vi "AES-Single-Round-Top.vi"(9 "state (_c) U64":u64[](array[numeric]) format="%.0x", 11 "key (_a)":u64[](array[numeric]) format="%.0x") -> (1 "state out (c) U64":u64[](array[numeric]) format="%.0x")   [LabVIEW 2017]
uses:
  AES-xtime.vi
panel:
  out "ADD_KEY":u8[](array[numeric]) format="%.0x"
  out "MIX_COLUMNS":u8[](array[numeric]) format="%.0x"
  out "SHIFT_ROWS":u8[](array[numeric]) format="%.0x"
  out "SUB_BYTES":u8[](array[numeric]) format="%.0x"
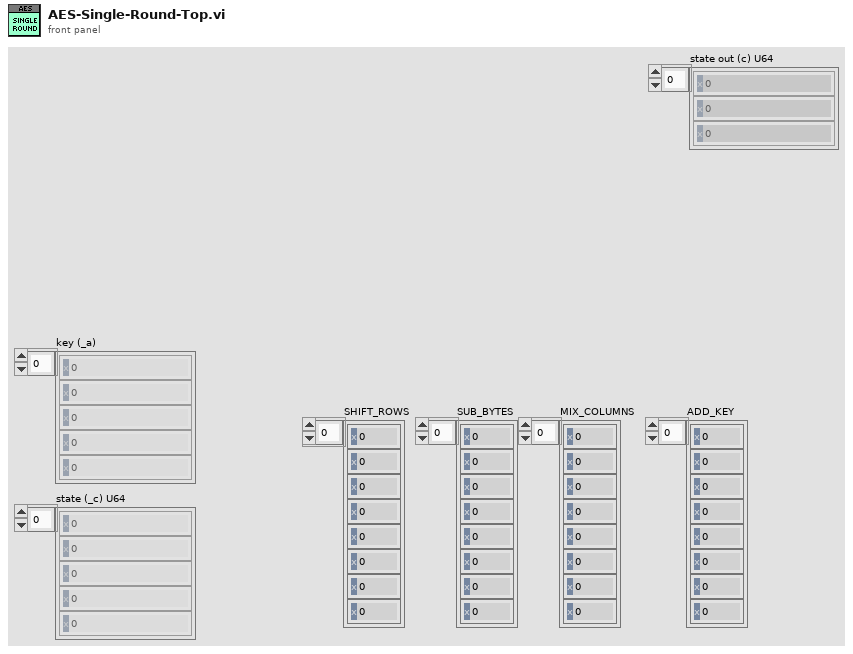
[diagram p1: front panel]
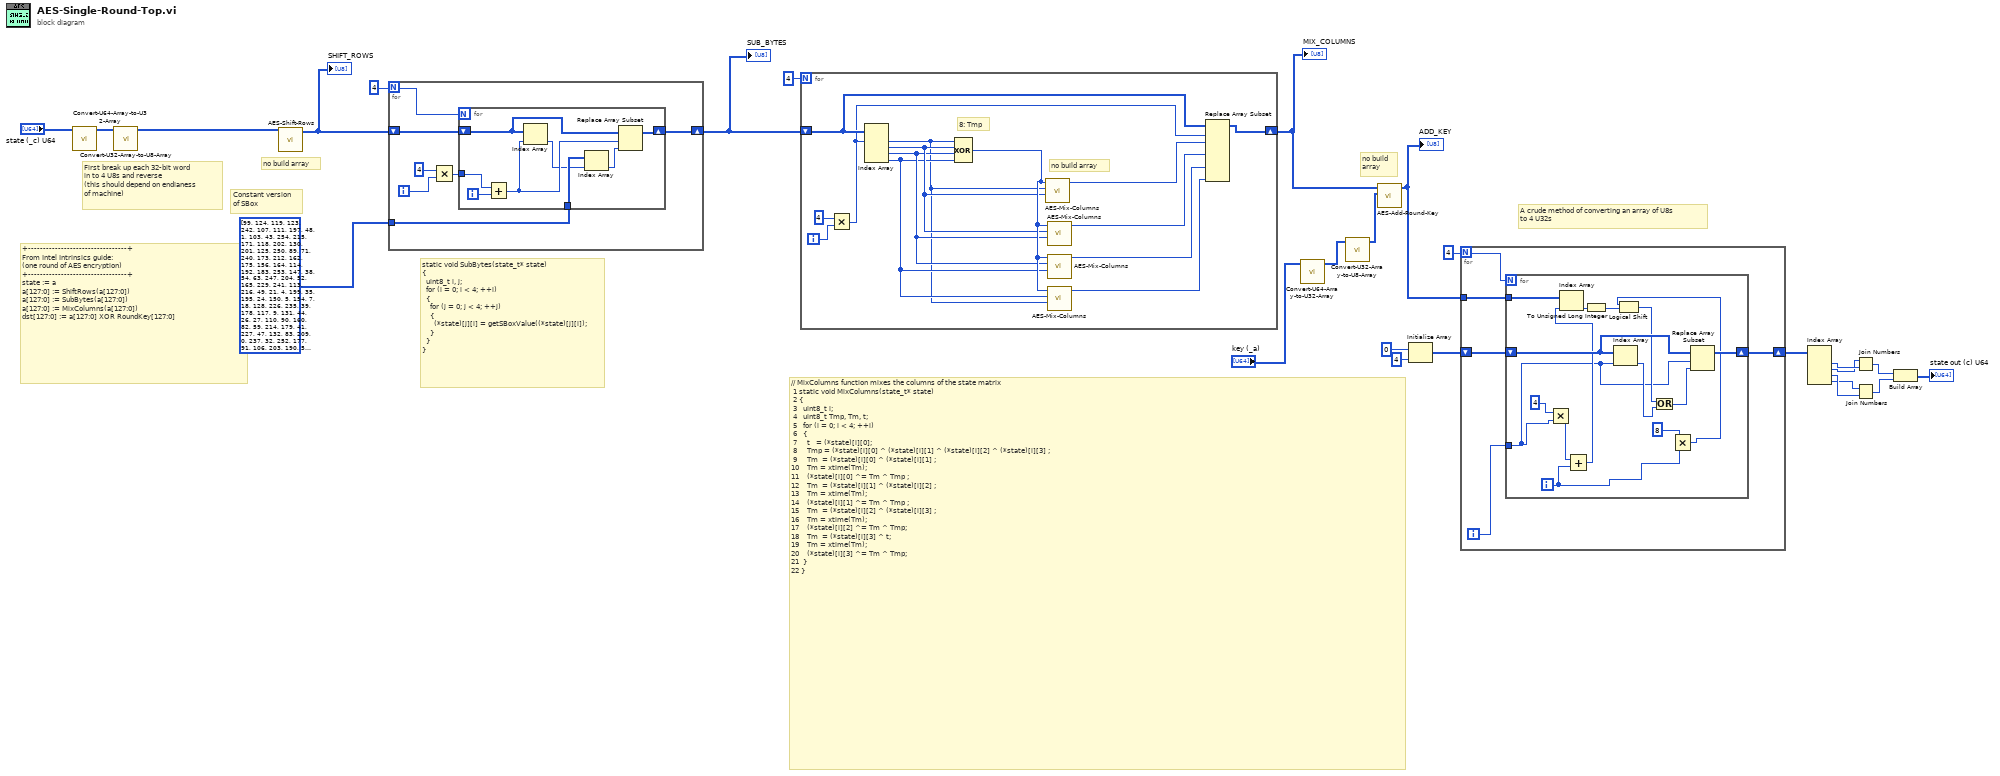
[diagram p0: block diagram]
diagram:
  # "A crude method of converting an array of U8s\nto 4 U32s"
  # "no build\narray"
  # "no build array"
  # "Constant version\nof SBox"
  # "// MixColumns function mixes the columns of the state matrix\n 1 static void MixColumns(state_t* state)\n 2 {\n 3   uint8_t i;\n 4   uint8_t Tmp, Tm, t;\n 5   for (i = 0; i < 4; ++i)\n 6   {  \n 7     t   = (*state)[i][0]; \n 8     Tmp = (*state)[i][0] ^ (*state)[i][1] ^ (*state)[i][2] ^ (*state)[i][3] ;\n 9     Tm  = (*state)[i][0] ^ (*state)[i][1] ;\n10    Tm = xtime(Tm);  \n11    (*state)[i][0] ^= Tm ^ Tmp ;\n12    Tm  = (*state)[i][1] ^ (*state)[i][2] ; \n13    Tm = xtime(Tm);  \n14    (*state)[i][1] ^= Tm ^ Tmp ;\n15    Tm  = (*state)[i][2] ^ (*state)[i][3] ;\n16    Tm = xtime(Tm);\n17    (*state)[i][2] ^= Tm ^ Tmp;\n18    Tm  = (*state)[i][3] ^ t;\n19    Tm = xtime(Tm);\n20    (*state)[i][3] ^= Tm ^ Tmp;\n21  }\n22 }"
  # "static void SubBytes(state_t* state)\n{\n  uint8_t i, j;\n  for (i = 0; i < 4; ++i)\n  {\n    for (j = 0; j < 4; ++j)\n    {\n      (*state)[j][i] = getSBoxValue((*state)[j][i]);\n    }\n  }\n}"
  # "First break up each 32-bit word\nin to 4 U8s and reverse\n(this should depend on endianess\nof machine)"
  # "+---------------------------------+\nFrom Intel Intrinsics guide:\n(one round of AES encryption)\n+---------------------------------+\nstate := a\na[127:0] := ShiftRows(a[127:0])\na[127:0] := SubBytes(a[127:0])\na[127:0] := MixColumns(a[127:0])\ndst[127:0] := a[127:0] XOR RoundKey[127:0]"
  n1 = call "Convert-U64-Array-to-U32-Array.vi"("2 x U64"="state (_c) U64") -> ("4 x U32"=w9:u32[])  [unwired: 10 in]
  n2 = call "Convert-U32-Array-to-U8-Array.vi"("state"=w9) -> ("Array"=w25:u8[])  [unwired: 10 in]
  n3 = call "AES-Shift-Rows.vi"("Data In"=w25) -> ("Data Out"=w23:u8[])  [unwired: 10 in]
  "SHIFT_ROWS" <- w23
  n4 = for {
    N: 4 -> [w32]
    shift-right: [w29] -> w21
    shift-left: w23 -> [w31]
    tunnel: u8[] [99, 124, 119, 123, 242, 107, 111, 197, 48, 1, 103, 43, 254, 215, 171, 118, 202, 130, 201, 125, 250, 89, 71, 240, 173, 212, 162, 175, 156, 164, 114, 192, 183, 253, 147, 38, 54, 63, 247, 204, 52, 165, 229, 241, 113, 216, 49, 21, 4, 199, 35, 195, 24, 150, 5, 154, 7, 18, 128, 226, 235, 39, 178, 117, 9, 131, 44, 26, 27, 110, 90, 160, 82, 59, 214, 179, 41, 227, 47, 132, 83, 209, 0, 237, 32, 252, 177, 91, 106, 203, 190, 57, 74, 76, 88, 207, 208, 239, 170, 251, 67, 77, 51, 133, 69, 249, 2, 127, 80, 60, 159, 168, 81, 163, 64, 143, 146, 157, 56, 245, 188, 182, 218, 33, 16, 255, 243, 210, 205, 12, 19, 236, 95, 151, 68, 23, 196, 167, 126, 61, 100, 93, 25, 115, 96, 129, 79, 220, 34, 42, 144, 136, 70, 238, 184, 20, 222, 94, 11, 219, 224, 50, 58, 10, 73, 6, 36, 92, 194, 211, 172, 98, 145, 149, 228, 121, 231, 200, 55, 109, 141, 213, 78, 169, 108, 86, 244, 234, 101, 122, 174, 8, 186, 120, 37, 46, 28, 166, 180, 198, 232, 221, 116, 31, 75, 189, 139, 138, 112, 62, 181, 102, 72, 3, 246, 14, 97, 53, 87, 185, 134, 193, 29, 158, 225, 248, 152, 17, 105, 217, 142, 148, 155, 30, 135, 233, 206, 85, 40, 223, 140, 161, 137, 13, 191, 230, 66, 104, 65, 153, 45, 15, 176, 84, 187, 22] ("Array") -> [w30]
    i -> [w28]
    n5 = Multiply(x=4, y=w28) -> (x*y=w26:i32)
    n6 = for {
      N: w32 -> [_]
      tunnel: w26 -> [w40]
      shift-right: [w33] -> w29
      shift-left: w31 -> [w38]
      tunnel: w30 -> [w36]
      i -> [w39]
      n7 = Add(x=w40, y=w39) -> (x+y=w37:i32)
      n8 = Index Array(array=w38, index=w37) -> (element=w35:u8)
      n9 = Index Array(array=w36, index=w35) -> (element=w34:u8)
      n10 = Replace Array Subset(array=w38, new element=w34, index=w37) -> (w33:u8[])
    }
  }
  "SUB_BYTES" <- w21
  n11 = for {
    N: 4 -> [_]
    shift-right: [w41] -> w20
    shift-left: w21 -> [w52]
    i -> [w53]
    # "no build array"
    # "8: Tmp"
    n12 = Multiply(x=4, y=w53) -> (x*y=w51:i32)
    n13 = Index Array(array=w52, index #1=w51) -> (element #1=w42:u8, element #2=w45:u8, element #3=w44:u8, element #4=w43:u8)  [unwired: 3 in]
    n14 = Compound Arithmetic op=XOR(w42, w45, w44, w43) -> (w46:u8)
    n15 = call "AES-Mix-Columns.vi"("state[i][y]"=w45, "state[i][x]"=w42, "Tmp"=w46) -> ("state[i][x]"=w50:u8)  [unwired: 8 in]
    n16 = call "AES-Mix-Columns.vi"("state[i][y]"=w44, "state[i][x]"=w45, "Tmp"=w46) -> ("state[i][x]"=w49:u8)  [unwired: 8 in]
    n17 = call "AES-Mix-Columns.vi"("state[i][y]"=w43, "state[i][x]"=w44, "Tmp"=w46) -> ("state[i][x]"=w48:u8)  [unwired: 8 in]
    n18 = call "AES-Mix-Columns.vi"("state[i][y]"=w42, "state[i][x]"=w43, "Tmp"=w46) -> ("state[i][x]"=w47:u8)  [unwired: 8 in]
    n19 = Replace Array Subset(array=w52, new element #1=w50, index #1=w51, new element #2=w49, new element #3=w48, new element #4=w47) -> (w41:u8[])  [unwired: 3 in]
  }
  "MIX_COLUMNS" <- w20
  n20 = call "Convert-U64-Array-to-U32-Array.vi"("2 x U64"="key (_a)") -> ("4 x U32"=w12:u32[])  [unwired: 10 in]
  n21 = call "Convert-U32-Array-to-U8-Array.vi"("state"=w12) -> ("Array"=w19:u8[])  [unwired: 10 in]
  n22 = call "AES-Add-Round-Key.vi"("Roundkey In"=w19, "Data In"=w20) -> ("Array Out"=w17:u8[])  [unwired: 9 in]
  "ADD_KEY" <- w17
  n23 = Initialize Array(u32 0 ("element"), 4 ("dimension size")) -> (w14:u32[])
  n24 = for {
    N: 4 -> [w59]
    tunnel: w17 -> [w57]
    shift-right: [w56] -> w8
    shift-left: w14 -> [w58]
    i -> [w55]
    n25 = for {
      N: w59 -> [_]
      tunnel: w55 -> [w61]
      shift-right: [w69] -> w56
      shift-left: w58 -> [w74]
      tunnel: w57 -> [w73]
      i -> [w66]
      n26 = Multiply(x=4, y=w61) -> (x*y=w60:i32)
      n27 = Add(x=w60, y=w66) -> (x+y=w72:i32)
      n28 = Index Array(array=w73, index=w72) -> (element=w68:u8)
      n29 = To Unsigned Long Integer(number=w68) -> (unsigned 32bit integer=w63:u32)
      n30 = Index Array(array=w74, index=w61) -> (element=w71:u32)
      n31 = Multiply(x=8, y=w66) -> (x*y=w64:i32)
      n32 = Logical Shift(y=w64, x=w63) -> (x << y=w67:u32)
      n33 = Or(x=w67, y=w71) -> (x .or. y?=w70:u32)
      n34 = Replace Array Subset(array=w74, new element=w70, index=w61) -> (w69:u32[])
    }
  }
  n35 = Index Array(array=w8) -> (element #1=w7:u32, element #2=w6:u32, element #3=w5:u32, element #4=w4:u32)  [unwired: 4 in]
  n36 = Join Numbers(hi=w6, lo=w7) -> ((hi.lo)=w3:u64)
  n37 = Join Numbers(hi=w4, lo=w5) -> ((hi.lo)=w2:u64)
  n38 = Build Array(w3, w2) -> (→"state out (c) U64":u64[])
